vi "Read Measurement.vi"(8 "error in":errorcluster, 10 "call id":T1, 11 "gRPCid in":T1) -> (0 "error out":errorcluster, 1 "measure success?":bool, 2 "measurement results":T2, 3 "gRPCid out":T1)   [LabVIEW 2021, in "Measurement Client Template.lvlib"]
uses:
  Measurement Client Template.lvlib
  <vilib>/gRPC/LabVIEW gRPC Library/Shared/grpcId.ctl
  controls/Measurement Results.ctl
  34829905-00c5-4e32-9a4f-e87a22ec28de.vi
  <vilib>/gRPC/LabVIEW gRPC Library/Server API/Translate Protobuf Error.vi
  <vilib>/AdvancedString/1D String Array to Delimited String.vi
  <vilib>/gRPC/LabVIEW gRPC Library/Server API/Server/Get Server DLL Path.vi
  <vilib>/gRPC/Generated APIs/ni/measurementlink/measurement/v2/Measurement Service Client V2/Measurement Service Client V2.lvlib
  <vilib>/gRPC/LabVIEW gRPC Library/grpc-lvsupport-release.lvlib
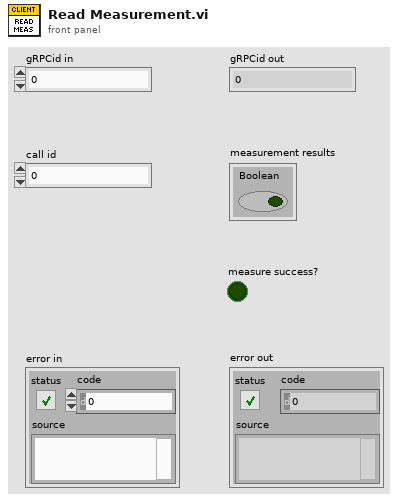
[diagram p1: front panel]
types:
  T1 = typedef "grpc-lvsupport-release.lvlib/grpcId.ctl" = u64
  T2 = typedef "Measurement Client Template.lvlib/Measurement Results.ctl" = cluster{"Boolean":bool}
  T3 = typedef "Measurement Service Client V2.lvlib/ni_measurementlink_measurement_v2_MeasureResponse.ctl" = cluster{"outputs":T4}
  T4 = typedef "Measurement Service Client V2.lvlib/google_protobuf_Any.ctl" = cluster{"type_url":string, "value":u8[]}
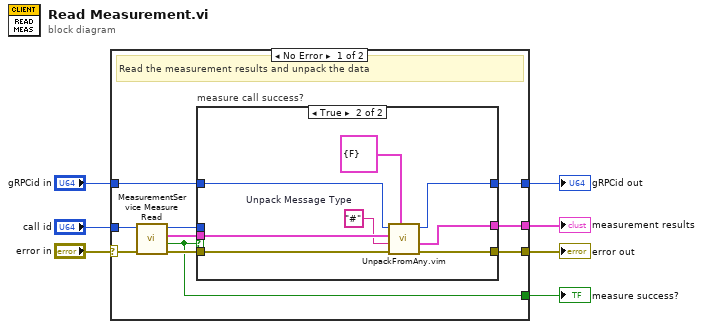
[diagram p0: block diagram]
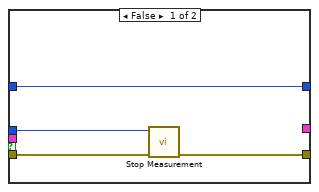
[diagram p2: hidden frame]
diagram:
  n1 = case shown="No Error" "error in" {
    selector: "error in" -> [w14 w30]
    tunnel: "gRPCid in" -> [w16 w31]
    tunnel: "call id" -> [w15 _]
    tunnel: [w13 _] -> w4
    tunnel: [w12 w31] -> w3
    tunnel: [w9 w30] -> w2
    tunnel: [w8 _] -> w1
    frame No Error {
      # "Read the measurement results and unpack the data"
      n2 = call <vilib>:"MeasurementService Measure Read.vi"("error in"=w14, "Call ID in"=w15) -> ("error out"=w11:errorcluster, "Success"=w8:bool, "Response Data"=w10:T3, "Call ID"=w17:T1)  [unwired: 6 in]
      n3 = case "measure call success?" shown="True" w8 {
        tunnel: w10 -> [_ w29]
        tunnel: [w19 w28] -> w9
        tunnel: w11 -> [w20 w27]
        tunnel: [w21 w25] -> w12
        tunnel: [_ w23] -> w13
        tunnel: w16 -> [w21 w22]
        tunnel: w17 -> [w18 _]
        frame False {
          n4 = call "Stop Measurement.vi"("error in"=w20, "call id"=w18) -> ("error out"=w19:errorcluster)  [unwired: 9 in]
        }
        frame True {
          w24 = "#"  # Unpack Message Type
          n5 = call "UnpackFromAny.vim"("Data Type"=T2 {"Boolean"=FALSE} ("measurement results"), "error in"=w27, "Message Type"=w24, "Any"=w29, "gRPCid in"=w22) -> ("error out"=w28:errorcluster, "Unpacked Value"=w23:T2, "gRPCid out"=w25:u64)  [unwired: 4 in]
        }
      }
    }
    frame Error {
      # "Pass"
    }
  }
  "measurement results" <- w4
  "gRPCid out" <- w3
  "error out" <- w2
  "measure success?" <- w1
